vi "Can Add Timing Channels.vi"(8 "error in":errorcluster, 11 "Node Ptr":T2 format="%.0x") -> (0 "error out":errorcluster, 3 "Action":T1)   [LabVIEW 2020, in "AIM ARINC 429 System Explorer.lvlib" / "Implementation.lvlib"]
uses:
  Implementation.lvlib
  <vilib>/NI VeriStand/Custom Device API/Custom Device Item Ref.ctl
  <vilib>/NI VeriStand/Custom Device API/Custom Device RTM Dependency.ctl
  <vilib>/NI VeriStand/Custom Device API/Custom Device API.lvlib
  Scripting/AIM/AIM ARINC 429 Scripting.lvlib
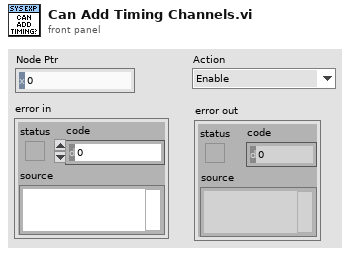
[diagram p1: front panel]
types:
  T1 = typedef "Custom Device API.lvlib/Custom Device RTM Dependency.ctl" = enum16{"Enable", "Disable", "Hide"}
  T2 = typedef "Custom Device API.lvlib/Custom Device Item Ref.ctl" = u64
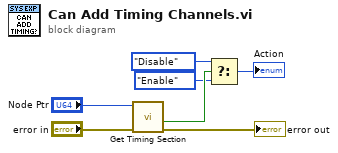
[diagram p0: block diagram]
diagram:
  n1 = call "Get Timing Section.vi"("error in"="error in", "custom device ref"="Node Ptr") -> ("error out"=→"error out":errorcluster, "Found"=w4:bool)  [unwired: 6 in, 2 out]
  n2 = Select(t=Custom_Device_RTM_Dependency."Disable" ("Action"), s=w4, f=Custom_Device_RTM_Dependency."Enable" ("Action")) -> (s? t:f=→"Action":T1)
